vi "constant vi validation.vi"(10 "New Constant vi name":string, 11 "Constant VI List":string[](array[string])) -> (3 "Proceed with Scripting":bool)   [LabVIEW 2020, in "ConstantErrorsMaker.lvlib"]
uses:
  ConstantErrorsMaker.lvlib
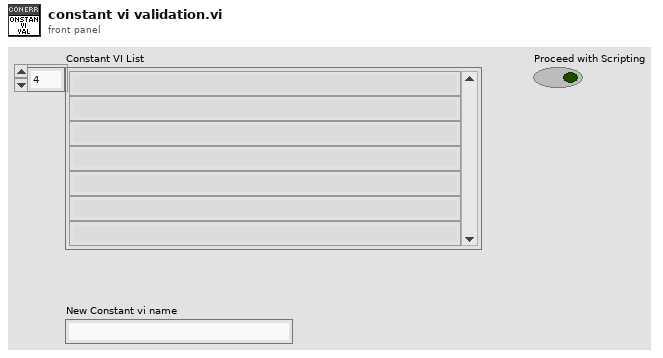
[diagram p1: front panel]
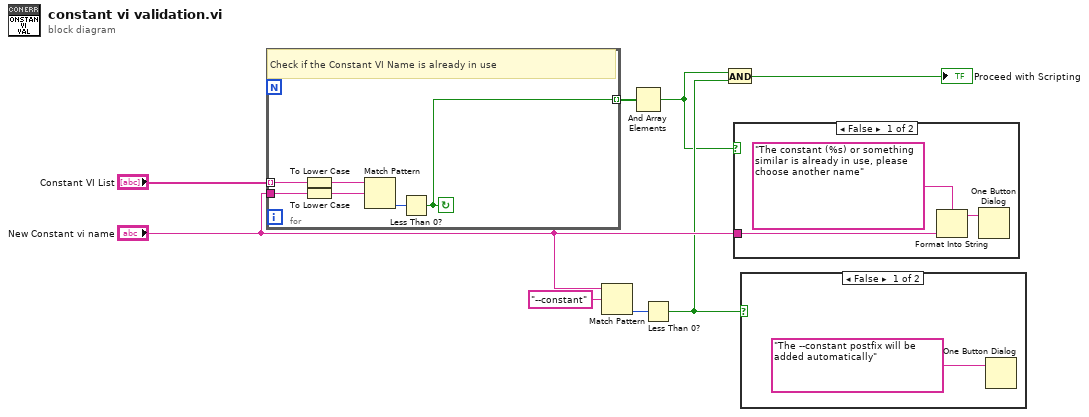
[diagram p0: block diagram]
diagram:
  n1 = for {
    tunnel: "Constant VI List" -> [w10] mode=indexing
    tunnel: "New Constant vi name" -> [w14]
    tunnel: [w12] -> w7 mode=indexing
    stop <- w12 continue-if-true
    # "Check if the Constant VI Name is already in use"
    n2 = To Lower Case(string=w10) -> (all lower case string=w9:string)
    n3 = To Lower Case(string=w14) -> (all lower case string=w11:string)
    n4 = Match Pattern(string=w9, regular expression=w11) -> (offset past match=w13:i32)  [unwired: 1 in, 3 out]
    n5 = Less Than 0?(x=w13) -> (x < 0?=w12:bool)
  }
  n6 = Match Pattern(string="New Constant vi name", regular expression="--constant") -> (offset past match=w5:i32)  [unwired: 1 in, 3 out]
  n7 = And Array Elements(Boolean array=w7) -> (logical AND=w2:bool)
  n8 = Less Than 0?(x=w5) -> (x < 0?=w3:bool)
  n9 = And(x=w2, y=w3) -> (x .and. y?=→"Proceed with Scripting":bool)
  n10 = case shown="False" w2 {
    tunnel: "New Constant vi name" -> [w16 _]
    frame False {
      n11 = Format Into String(format string="The constant (%s) or something similar is already in use, please choose another name", w16) -> (resulting string=w17:string)  [unwired: 2 in, 1 out]
      n12 = One Button Dialog(message=w17) -> ()  [unwired: 1 in, 1 out]
    }
    frame True {
    }
  }
  n13 = case shown="False" w3 {
    frame False {
      n14 = One Button Dialog(message="The --constant postfix will be added automatically" ("format string")) -> ()  [unwired: 1 in, 1 out]
    }
    frame True {
    }
  }
